vi "Remove ECU Event RTM Dependency.vi"(8 "error in (no error)":errorcluster, 9 "Menu hierarchy in":string[](array[string]), 11 "Node Ptr":u64 format="%.0x") -> (0 "error out":errorcluster, 1 "Menu hierarchy out":string[](array[string]), 3 "Action":T1)   [LabVIEW 2011, in "Engine Simulation Custom Device.lvlib"]
uses:
  Engine Simulation Custom Device.lvlib
  <vilib>/NI Veristand/Custom Device API/Custom Device API.lvlib
  Engine Simulation Global.vi
  <vilib>/NI Veristand/Custom Device API/Get Item Property (Variant).vi
  <vilib>/NI Veristand/Custom Device API/Custom Device RTM Dependency.ctl
  TypeDefs/ECUEventComp.ctl
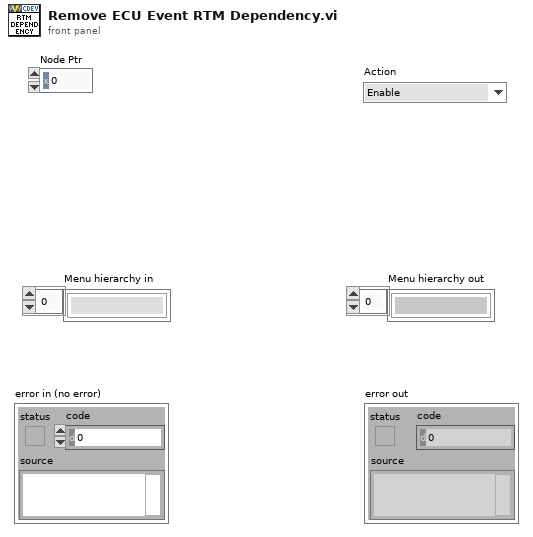
[diagram p1: front panel]
types:
  T1 = typedef "Custom Device API.lvlib/Custom Device RTM Dependency.ctl" = enum16{"Enable", "Disable", "Hide"}
  T2 = typedef "Engine Simulation Custom Device.lvlib/ECUEventComp.ctl" = cluster{"Name":string, "Time Duration":bool, "Start Angle":bool, "End Angle":bool, "Angle Duration":bool}
  T3 = typedef "Custom Device API.lvlib/Custom Device Item Ref.ctl" = u64
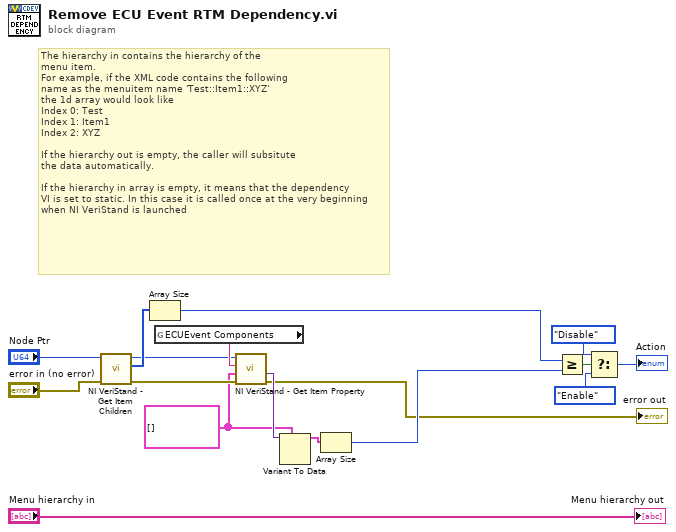
[diagram p0: block diagram]
diagram:
  w3 = T2[] []
  # "The hierarchy in contains the hierarchy of the\nmenu item.\nFor example, if the XML code contains the following\nname as the menuitem name 'Test::Item1::XYZ'\nthe 1d array would look like\nIndex 0: Test\nIndex 1: Item1\nIndex 2: XYZ\n\nIf the hierarchy out is empty, the caller will subsitute\nthe data automatically.\n\nIf the hierarchy in array is empty, it means that the dependency\nVI is set to static. In this case it is called once at the very beginning\nwhen NI VeriStand is launched"
  n1 = call <vilib>:"NI VeriStand - Get Item Children.vi"("error in (no error)"="error in (no error)", "Item Ref in"="Node Ptr") -> ("error out"=w9:errorcluster, "Child Refs"=w15:T3[], "Item Ref out"=w10:T3)  [unwired: 6 in, 1 out]
  n2 = Array Size(array=w15) -> (size(s)=w8:i32)
  n3 = global read "Engine Simulation Global.vi" "ECUEvent Components"() -> (w13:string)
  n4 = call-poly <vilib>:"NI VeriStand - Get Item Property.vi"("error in (no error)"=w9, "Default Value"=w3, "Property Name"=w13, "Item Ref in"=w10) -> ("error out"=→"error out":errorcluster, "Value"=w12:variant)  [unwired: 4 in, 2 out]
  n5 = Variant To Data(type=w3, Variant=w12) -> (data=w11:T2[])  [unwired: 1 in, 1 out]
  n6 = Array Size(array=w11) -> (size(s)=w2:i32)
  n7 = Greater Or Equal?(x=w8, y=w2) -> (x >= y?=w7:bool)
  n8 = Select(t=Custom_Device_RTM_Dependency."Disable" ("Action"), s=w7, f=Custom_Device_RTM_Dependency."Enable" ("Action")) -> (s? t:f=→"Action":T1)
  "Menu hierarchy out" <- "Menu hierarchy in"
